vi "Get Length.vi"(8 "error in (no error)":errorcluster, 11 "Graph Manager in":refnum<class "Graph Manager.lvclass">) -> (0 "error out":errorcluster, 2 "length":i32, 3 "Graph Manager out":refnum<class "Graph Manager.lvclass">)   [LabVIEW 2016, in "Graph Manager.lvclass"]
uses:
  Graph Manager.lvclass
  Graph Manager.lvclass/Graph Manager.ctl
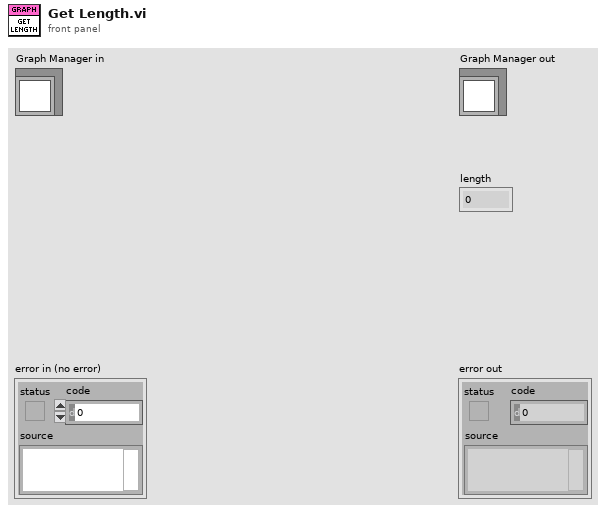
[diagram p1: front panel]
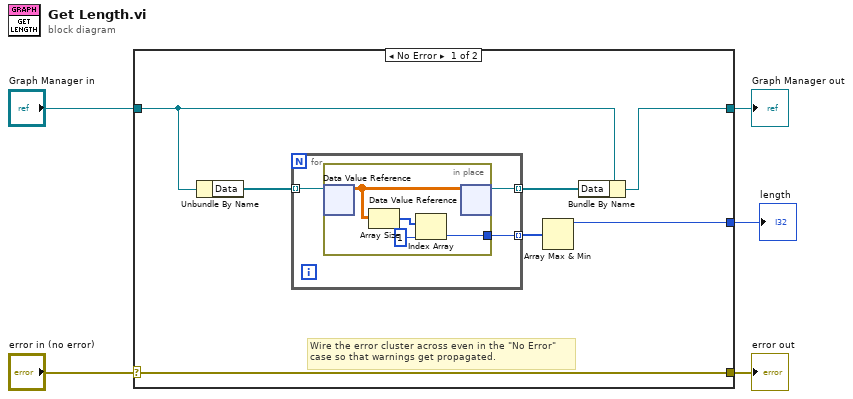
[diagram p0: block diagram]
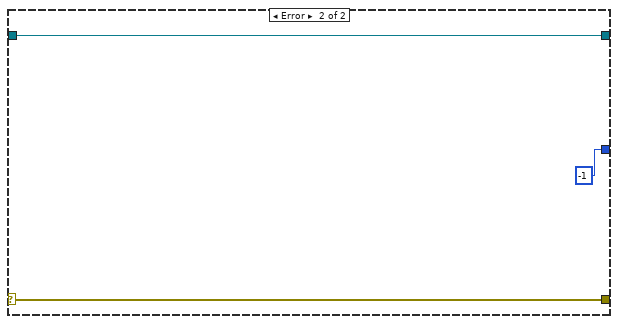
[diagram p2: hidden frame]
diagram:
  n1 = case shown="No Error" "error in (no error)" {
    selector: "error in (no error)" -> [w12 w22]
    tunnel: [w12 w22] -> w4
    tunnel: [w9 w21] -> w2
    tunnel: "Graph Manager in" -> [w10 w21]
    tunnel: [w6 -1] -> w1
    frame No Error {
      # "Wire the error cluster across even in the \"No Error\"\ncase so that warnings get propagated."
      n2 = Unbundle By Name(w10) -> ("Data"=w11:refnum<data-value>[])
      n3 = for {
        tunnel: w11 -> [w15] mode=indexing
        tunnel: [w14] -> w8 mode=indexing
        tunnel: [w13] -> w7 mode=indexing
        n4 = in-place {
          in-place-border: [w16] -> w13
          n5 = in-place-dvr #1(w15) -> (w19:dbl[][])  [unwired: 1 out]
          n6 = Array Size(array=w19) -> (size(s)=w18:i32[])
          n7 = Index Array(array=w18, index=1) -> (element=w16:i32)
          n8 = in-place-dvr #1(w19) -> (w14:refnum<data-value>)  [unwired: 1 out]
        }
      }
      n9 = Array Max & Min(array=w7) -> (max value=w6:i32)  [unwired: 3 out]
      n10 = Bundle By Name(cluster=w10, "Data"=w8) -> (w9:refnum<class "Graph Manager.lvclass">)
    }
    frame Error {
    }
  }
  "error out" <- w4
  "Graph Manager out" <- w2
  "length" <- w1
